vi "bomba2.vi"() -> ()   [LabVIEW 2020]
uses:
  <vilib>/Instr/_visa.llb/VISA Configure Serial Port (Instr).vi
panel:
  out "read buffer":string
  out "return count 2":u32
  in  "baud rate (9600)":u32=9600
  in  "VISA resource name":refnum<visa-resource-name>
  out "concatenated string":string
  out "F-format string":string
  out "return count":u32
  in  "stop":bool
  in  "Velocidad de la bomba":u8(slide) scale=0.0..255.0
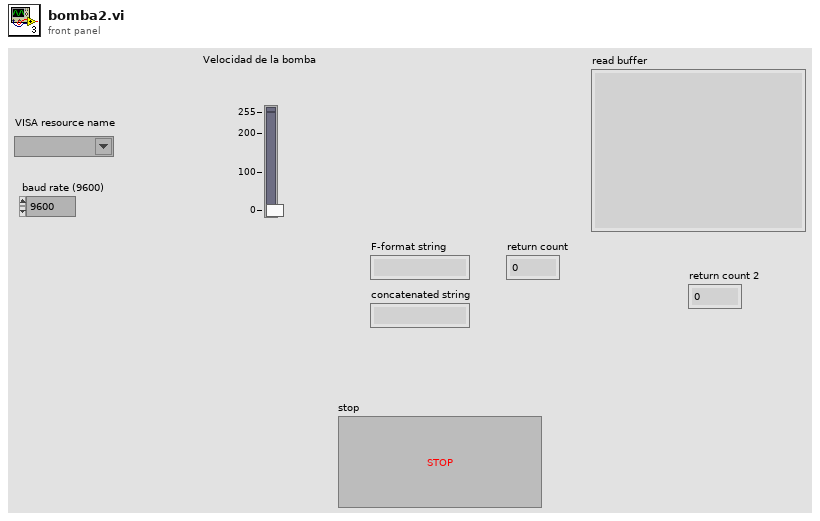
[diagram p1: front panel]
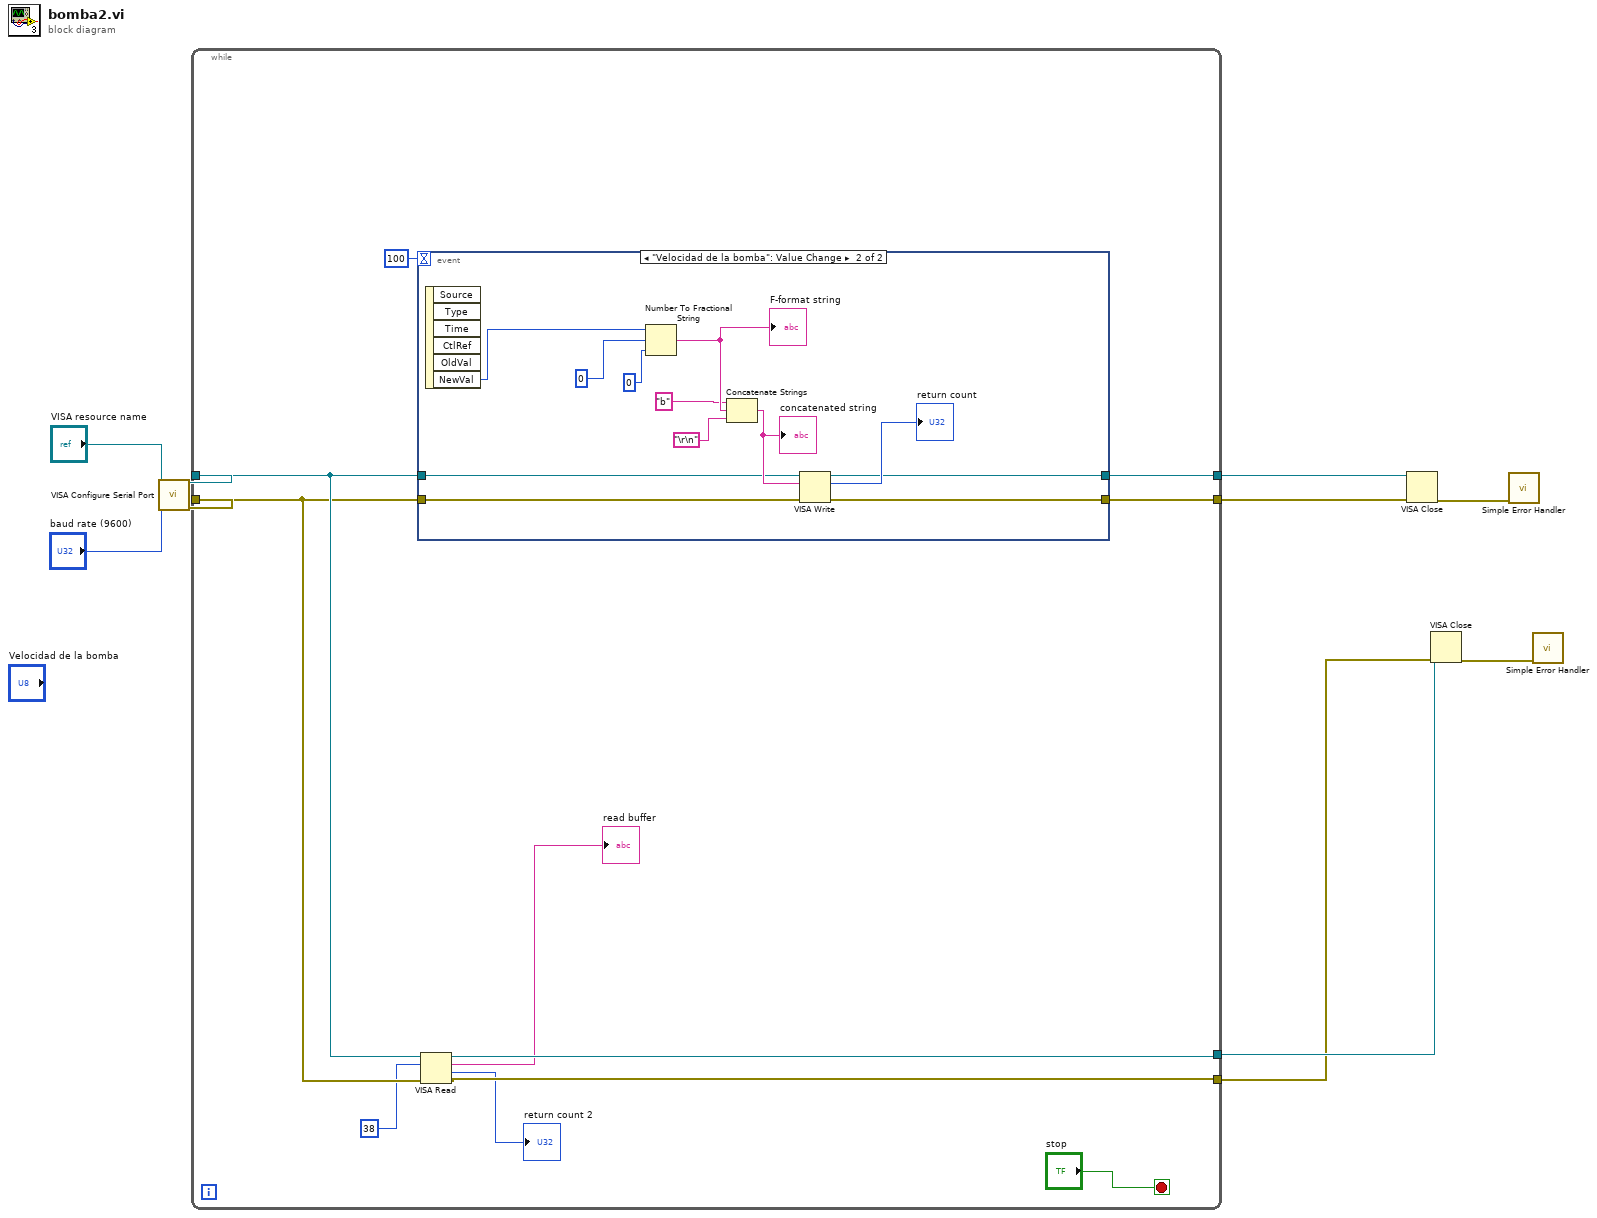
[diagram p0: block diagram]
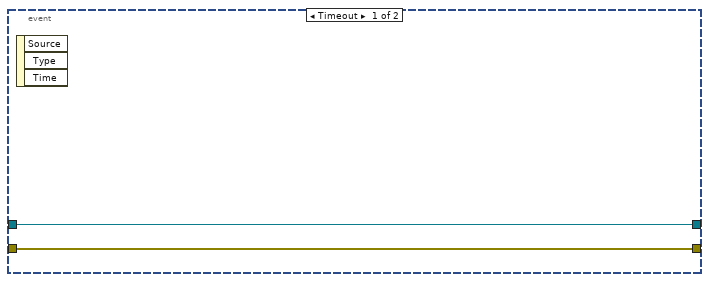
[diagram p2: hidden frame]
diagram:
  n1 = call-poly "VISA Configure Serial Port"("VISA resource name"="VISA resource name", "baud rate (9600)"="baud rate (9600)") -> ("VISA resource name out"=w9:refnum<visa-resource-name>, "error out"=w10:errorcluster)  [unwired: 12 in]
  n2 = while {
    tunnel: w10 -> [w17]
    tunnel: w9 -> [w18]
    tunnel: [w20] -> w6
    tunnel: [w19] -> w5
    tunnel: [w15] -> w2
    tunnel: [w14] -> w1
    stop <- "stop" stop-if-true
    n3 = event shown="[1] \"Velocidad de la bomba\": Value Change" {
      selector: _ -> [_ _]
      dyn-events: _ -> [_ _]
      timeout: 100 -> [_ _]
      tunnel: w17 -> [w22 w27]
      tunnel: w18 -> [w23 w26]
      tunnel: [w23 w25] -> w20
      tunnel: [w22 w24] -> w19
      event Timeout {
        n4 = event-data() -> ()  [unwired: 1 in, 3 out]
      }
      event "Velocidad de la bomba": Value Change {
        n5 = event-data() -> ("NewVal"=w28:u8)  [unwired: 1 in, 5 out]
        n6 = Number To Fractional String(number=w28, width (-)=i16 0, precision (6)=i16 0) -> (F-format string=w30:string)  [unwired: 1 in]
        "F-format string" <- w30
        n7 = Concatenate Strings("b" ("string"), w30, "\r\n") -> (w34:string)
        "concatenated string" <- w34
        n8 = VISA Write(VISA resource name=w26, write buffer=w34, error in (no error)=w27) -> (VISA resource name out=w25:refnum<visa-resource-name>, return count=→"return count":u32, error out=w24:errorcluster)
      }
    }
    n9 = VISA Read(VISA resource name=w18, byte count=u32 38, error in (no error)=w17) -> (VISA resource name out=w15:refnum<visa-resource-name>, read buffer=→"read buffer":string, return count=→"return count 2":u32, error out=w14:errorcluster)
  }
  n10 = VISA Close(VISA resource name=w6, error in (no error)=w5) -> (error out=w4:errorcluster)
  n11 = VISA Close(VISA resource name=w2, error in (no error)=w1) -> (error out=w3:errorcluster)
  n12 = call <vilib>:"Simple Error Handler.vi"("error in (no error)"=w4) -> ()  [unwired: 4 in, 5 out]
  n13 = call <vilib>:"Simple Error Handler.vi"("error in (no error)"=w3) -> ()  [unwired: 4 in, 5 out]
